vi "Copy Paste Time in Seconds.vi"() -> ()   [LabVIEW 2017]
panel:
  out "COPY PASTA":string
  out "Current Time in Seconds":u64 format="%012x"
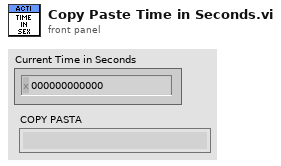
[diagram p1: front panel]
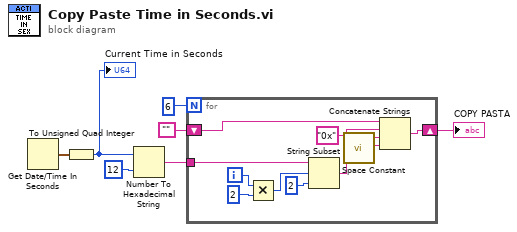
[diagram p0: block diagram]
diagram:
  n1 = Get Date/Time In Seconds() -> (seconds since 1Jan1904=w7:timestamp)
  n2 = To Unsigned Quad Integer(1:w7) -> (0:w6:u64)
  "Current Time in Seconds" <- w6
  n3 = Number To Hexadecimal String(1:i16 12 ("width (-)"), 2:w6) -> (0:w5:string)
  n4 = for {
    N: 6 -> [_]
    tunnel: w5 -> [w16]
    shift-right: [w8] -> w1
    shift-left: "" -> [w9]
    i -> [w14]
    n5 = Multiply(x=w14, y=2) -> (x*y=w13:i32)
    n6 = String Subset(string=w16, offset (0)=w13, length (rest)=2 ("length (rest)")) -> (substring=w12:string)
    n7 = call <vilib>:"Space Constant.vi"() -> ("String"=w10:string)
    n8 = Concatenate Strings(w9, "0x" ("string"), w12, w10) -> (w8:string)
  }
  "COPY PASTA" <- w1
